vi "RVHR - Get Image.vi"(4 "Scale Factor":dbl=10.0 format="%#_13g", 6 "Filename _L":string[](array[string]), 8 "error in (no error)":errorcluster, 9 "Image #":u8, 10 "Left Image Folder":path, 11 "Image":refnum<vi>) -> (0 "error out":errorcluster, 2 "Rectangle":T1)   [LabVIEW 2024]
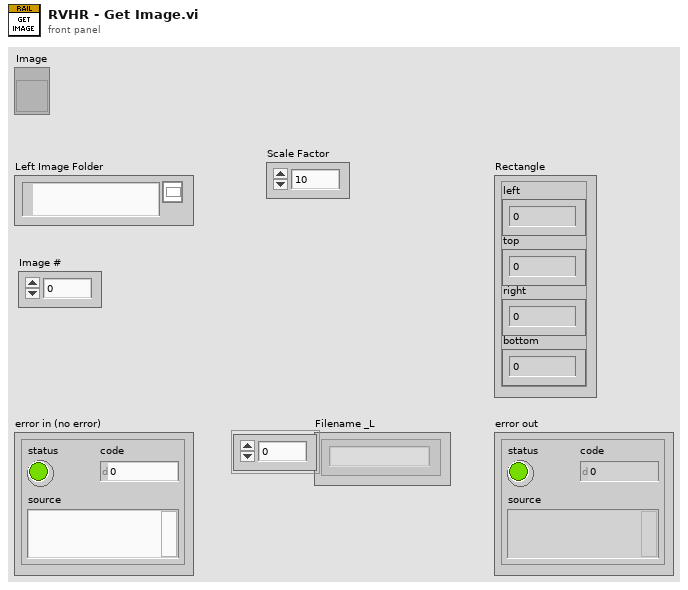
[diagram p1: front panel]
types:
  T1 = cluster{"left":i16, "top":i16, "right":i16, "bottom":i16}
  T2 = typedef "imagedata.ctl" = cluster{"image type":i32, "image depth":i32, "image":u8[], "mask":u8[], "colors":u32[], "Rectangle":cluster{"left":i16, "top":i16, "right":i16, "bottom":i16}}
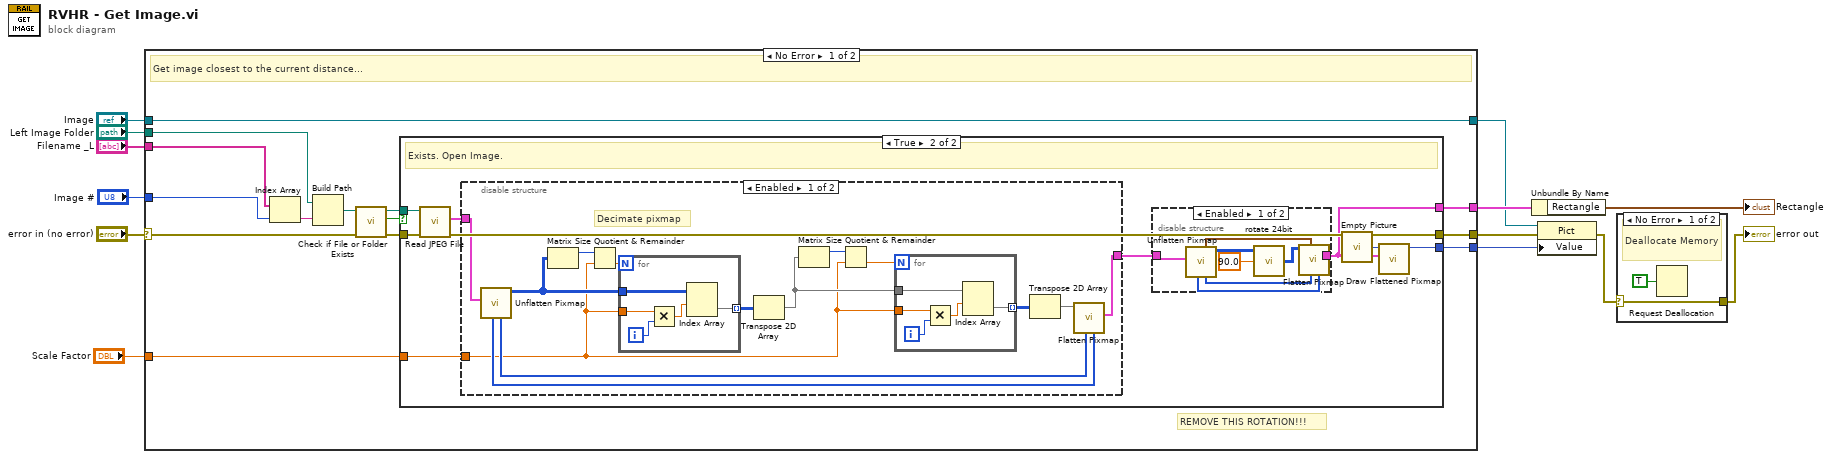
[diagram p0: block diagram]
diagram:
  n1 = case shown="No Error" "error in (no error)" {
    selector: "error in (no error)" -> [w26 w73]
    tunnel: [w27 _] -> w8
    tunnel: [w25 w73] -> w10
    tunnel: [w24 w72] -> w7
    tunnel: "Image" -> [w24 w72]
    tunnel: "Left Image Folder" -> [w21 _]
    tunnel: "Filename _L" -> [w23 _]
    tunnel: [w16 _] -> w9
    tunnel: "Scale Factor" -> [w15 _]
    tunnel: "Image #" -> [w14 _]
    frame No Error {
      # "REMOVE THIS ROTATION!!!"
      # "Get image closest to the current distance..."
      n2 = Index Array(array=w23, index=w14) -> (element=w22:string)
      n3 = Build Path(base path=w21, name or relative path=w22) -> (appended path=w20:path)
      n4 = call <vilib>:"Check if File or Folder Exists.vi"("error in (no error)"=w26, "path"=w20) -> ("error out"=w19:errorcluster, "file or folder exists?"=w17:bool, "dup path"=w18:path)  [unwired: 7 in]
      n5 = case shown="True" w17 {
        tunnel: [w28 w34] -> w25
        tunnel: w18 -> [_ w37]
        tunnel: w19 -> [w28 w36]
        tunnel: [_ w32] -> w16
        tunnel: [_ w33] -> w27
        tunnel: w15 -> [_ w29]
        frame False {
        }
        frame True {
          # "Exists. Open Image."
          n6 = call <vilib>:"Read JPEG File.vi"("error in (no error)"=w36, "path to JPEG file"=w37) -> ("error out"=w34:errorcluster, "image data"=w31:T2)  [unwired: 7 in, 1 out]
          n7 = disable-structure shown="Enabled" {
            disable-tunnel: w31 -> [w51 w62]
            disable-tunnel: [w41 w62] -> w30
            disable-tunnel: w29 -> [w38 _]
            frame Enabled {
              # "Decimate pixmap"
              n8 = call <vilib>:"Unflatten Pixmap.vi"("image data"=w51) -> ("24-bit pixmap"=w48:u32[][], "colors"=w39:u32[], "mask"=w40:u8[])  [unwired: 4 in, 4 out]
              n9 = Matrix Size(0:w48) -> (1:w50:i32)  [unwired: 1 out]
              n10 = Quotient & Remainder(x=w50, y=w38) -> (floor(x/y)=w49:dbl)  [unwired: 1 out]
              n11 = for {
                N: w49 -> [_]
                tunnel: w48 -> [w58]
                tunnel: w38 -> [w60]
                tunnel: [w57] -> w47 mode=indexing
                i -> [w61]
                n12 = Multiply(x=w60, y=w61) -> (x*y=w59:dbl)
                n13 = Index Array(array=w58, index (row)=w59) -> (element=w57:u32[])  [unwired: 1 in]
              }
              n14 = Transpose 2D Array(2D array=w47) -> (transposed array=w43:u32[][])
              n15 = Matrix Size(0:w43) -> (1:w46:i32)  [unwired: 1 out]
              n16 = Quotient & Remainder(x=w46, y=w38) -> (floor(x/y)=w45:dbl)  [unwired: 1 out]
              n17 = for {
                N: w45 -> [_]
                tunnel: w43 -> [w53]
                tunnel: w38 -> [w55]
                tunnel: [w52] -> w44 mode=indexing
                i -> [w56]
                n18 = Multiply(x=w55, y=w56) -> (x*y=w54:dbl)
                n19 = Index Array(array=w53, index (row)=w54) -> (element=w52:u32[])  [unwired: 1 in]
              }
              n20 = Transpose 2D Array(2D array=w44) -> (transposed array=w42:u32[][])
              n21 = call <vilib>:"Flatten Pixmap.vi"("mask"=w40, "colors"=w39, "24-bit pixmap"=w42) -> ("image data"=w41:T2)  [unwired: 8 in]
            }
            frame Disabled {
            }
          }
          n22 = disable-structure shown="Enabled" {
            disable-tunnel: w30 -> [w67 w71]
            disable-tunnel: [w66 w71] -> w32
            frame Enabled {
              n23 = call <vilib>:"Unflatten Pixmap.vi"("image data"=w67) -> ("24-bit pixmap"=w64:u32[][], "colors"=w69:u32[], "top left"=w70:cluster{"x":i16, "y":i16}, "mask"=w68:u8[])  [unwired: 4 in, 3 out]
              n24 = call "rotate 24bit.vi"("Rotation Angle (degrees)"=90.0, "Pixmap"=w64) -> ("Rotated Pixmap"=w63:u32[][])  [unwired: 2 in]
              n25 = call <vilib>:"Flatten Pixmap.vi"("mask"=w68, "colors"=w69, "top left"=w70, "24-bit pixmap"=w63) -> ("image data"=w66:T2)  [unwired: 7 in]
            }
            frame Disabled {
            }
          }
          n26 = call "Empty Picture"() -> ("empty picture"=w35:picture)
          n27 = call <vilib>:"Draw Flattened Pixmap.vi"("image data"=w32, "picture"=w35) -> ("new picture"=w33:picture)  [unwired: 7 in]
        }
      }
    }
    frame Error {
    }
  }
  n28 = Unbundle By Name(w9) -> ("Rectangle"=→"Rectangle":T1)
  n29 = property class="Pict"(reference=w7, error in=w10, "Value"=w8) -> (error out=w3:errorcluster)  [unwired: 1 out]
  n30 = case shown="No Error" w3 {
    selector: w3 -> [w74 w76]
    tunnel: [w74 w76] -> w2
    frame No Error {
      # "Deallocate Memory"
      n31 = Request Deallocation(TRUE ("flag")) -> ()
    }
    frame Error {
    }
  }
  "error out" <- w2
